vi "move files to target folder.vi"(8 "error in":errorcluster, 9 "overwrite (F)":bool, 10 "files":path[](array[path])=[path "C:/Users/Benjamin/Desktop/Test Folders/Folder odd/file 1.txt", path "C:/Users/Benjamin/Desktop/Test Folders/Folder odd/file 3.txt", path "C:/Users/Benjamin/Desktop/Test Folders/Folder odd/file 5.txt", path "C:/Users/Benjamin/Desktop/Test Folders/Folder odd/file 7.txt"], 11 "target folder":path=path "C:/Users/Benjamin/Desktop/Destination Folder") -> (0 "error out":errorcluster, 2 "new file paths":path[](array[path]), 3 "target folder duplicate":path)   [LabVIEW 2014]
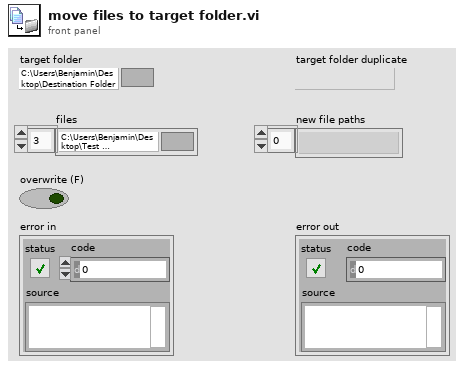
[diagram p1: front panel]
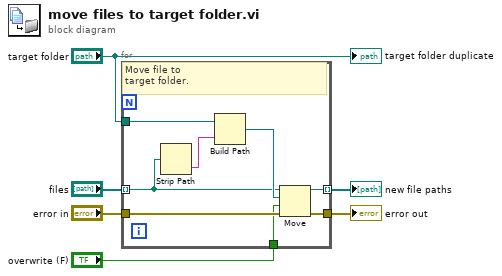
[diagram p0: block diagram]
diagram:
  n1 = for {
    tunnel: "files" -> [w8] mode=indexing
    tunnel: "target folder" -> [w14]
    tunnel: "error in" -> [w12]
    tunnel: [w11] -> w5
    tunnel: "overwrite (F)" -> [w10]
    tunnel: [w9] -> w3 mode=indexing
    # "Move file to \ntarget folder."
    n2 = Strip Path(path=w8) -> (name=w7:string)  [unwired: 1 out]
    n3 = Build Path(base path=w14, name or relative path=w7) -> (appended path=w13:path)
    n4 = Move(source path=w8, error in=w12, 9:w10, 10:w13) -> (error out=w11:errorcluster, 3:w9:path)  [unwired: 1 in, 1 out]
  }
  "error out" <- w5
  "new file paths" <- w3
  "target folder duplicate" <- "target folder"
